vi "GetPoutParameters.vi"(8 "error in (no error)":errorcluster, 11 "Motor Info":T3) -> (0 "error out":errorcluster, 1 "full load [kW]":dbl, 2 "additional efficiency information":T2(array[cluster]), 3 "nameplate information":T1(array[cluster]))   [LabVIEW 2017, in "McsaAnalysisFunctions.lvlib"]
uses:
  <vilib>/addons/InsightCM/Utilities/Analysis/MCSA/McsaAnalysisFunctions.lvlib
  <vilib>/addons/InsightCM/Utilities/Analysis/MCSA/controls/McsaMotor.ctl
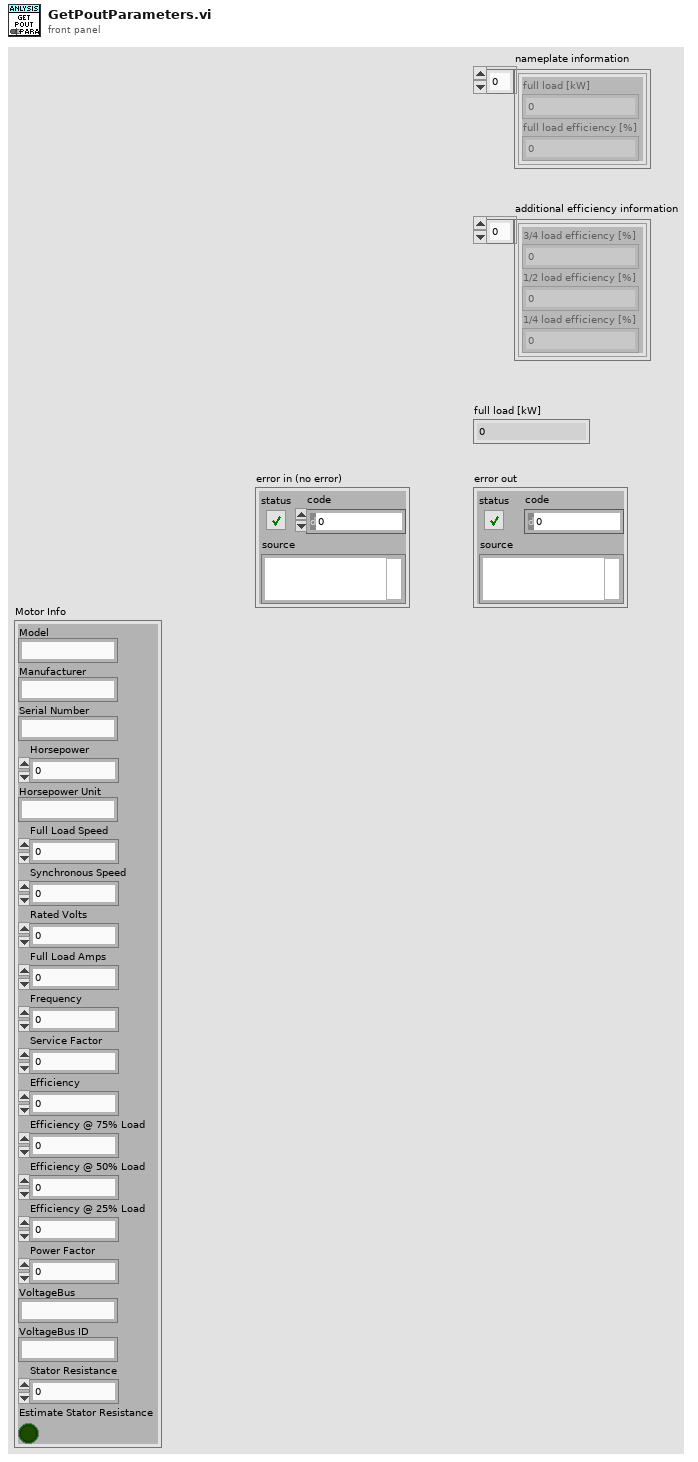
[diagram p1: front panel]
types:
  T1 = cluster{"full load [kW]":dbl, "full load efficiency [%]":dbl}[]
  T2 = cluster{"3/4 load efficiency [%]":dbl, "1/2 load efficiency [%]":dbl, "1/4 load efficiency [%]":dbl}[]
  T3 = typedef "McsaAnalysisFunctions.lvlib/McsaMotor.ctl" = cluster{"Model":string, "Manufacturer":string, "Serial Number":string, "Horsepower":dbl, "Horsepower Unit":string, "Full Load Speed":dbl, "Synchronous Speed":dbl, "Rated Volts":dbl, "Full Load Amps":dbl, "Frequency":dbl, "Service Factor":dbl, "Efficiency":dbl, "Efficiency @ 75% Load":dbl, "Efficiency @ 50% Load":dbl, "Efficiency @ 25% Load":dbl, "Power Factor":dbl, "VoltageBus":string, "VoltageBus ID":string, "Stator Resistance":dbl, "Estimate Stator Resistance":bool}
  T4 = cluster{"full load [kW]":dbl, "full load efficiency [%]":dbl}
  T5 = cluster{"3/4 load efficiency [%]":dbl, "1/2 load efficiency [%]":dbl, "1/4 load efficiency [%]":dbl}
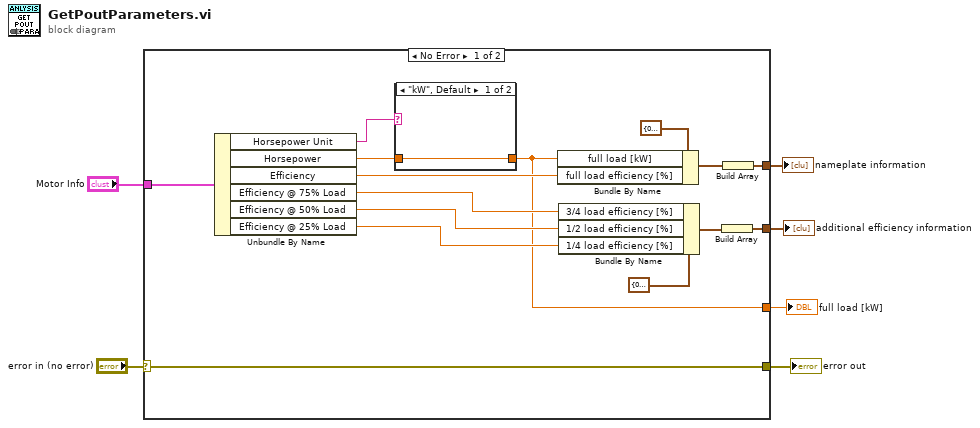
[diagram p0: block diagram]
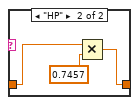
[diagram p2: hidden frame]
diagram:
  n1 = case shown="No Error" "error in (no error)" {
    selector: "error in (no error)" -> [w7 w26]
    tunnel: "Motor Info" -> [w21 _]
    tunnel: [w11 _] -> w5
    tunnel: [w9 _] -> w4
    tunnel: [w8 _] -> w3
    tunnel: [w7 w26] -> w1
    frame No Error {
      n2 = Unbundle By Name(w21) -> ("Horsepower Unit"=w18:string, "Horsepower"=w17:dbl, "Efficiency"=w19:dbl, "Efficiency @ 75% Load"=w15:dbl, "Efficiency @ 50% Load"=w14:dbl, "Efficiency @ 25% Load"=w13:dbl)
      n3 = case shown="\"kW\", Default" w18 {
        tunnel: [w22 w24] -> w8
        tunnel: w17 -> [w22 w25]
        frame "kW", Default {
        }
        frame "HP" {
          n4 = Multiply(x=w25, y=0.7457) -> (x*y=w24:dbl)
        }
      }
      n5 = Bundle By Name(cluster=T4 {"full load [kW]"=0.0, "full load efficiency [%]"=0.0} ("nameplate information"), "full load [kW]"=w8, "full load efficiency [%]"=w19) -> (w12:T4)
      n6 = Bundle By Name(cluster=T5 {"3/4 load efficiency [%]"=0.0, "1/2 load efficiency [%]"=0.0, "1/4 load efficiency [%]"=0.0} ("additional efficiency information"), "3/4 load efficiency [%]"=w15, "1/2 load efficiency [%]"=w14, "1/4 load efficiency [%]"=w13) -> (w10:T5)
      n7 = Build Array(w10) -> (w9:T2)
      n8 = Build Array(w12) -> (w11:T1)
    }
    frame Error {
    }
  }
  "error out" <- w1
  "additional efficiency information" <- w4
  "nameplate information" <- w5
  "full load [kW]" <- w3
